vi "LEBITplc.ParseMin&MaxArray.vi"(2 "Min&MaxArray":string[][](array[string])) -> (15 "MinSetValue":dbl[](array[numeric]), 16 "MaxSetValue":dbl[](array[numeric]), 17 "SetValueInfoServiceId":i32[](array[numeric]))   [LabVIEW 2014, in "LEBITplc.lvlib"]
uses:
  LEBITplc.lvlib
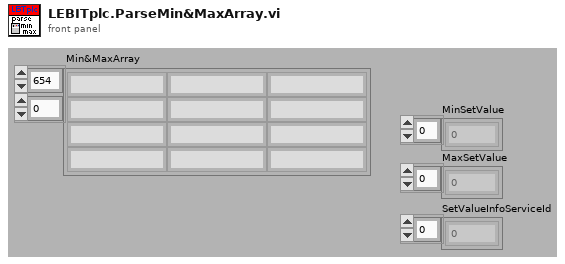
[diagram p1: front panel]
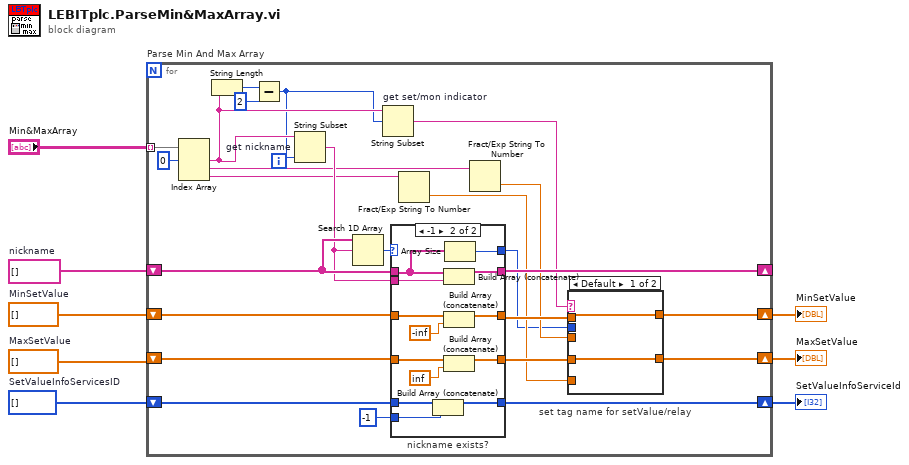
[diagram p0: block diagram]
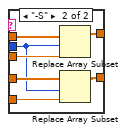
[diagram p3: hidden frame]
diagram:
  w4 = i32[] []  # SetValueInfoServicesID
  w5 = dbl[] []  # MaxSetValue
  w6 = dbl[] []  # MinSetValue
  w8 = string[] []  # nickname
  n1 = for "Parse Min And Max Array" {
    tunnel: "Min&MaxArray" -> [w33] mode=indexing
    shift-right: [w22] -> _
    shift-left: w8 -> [w26]
    shift-right: [w21] -> w2
    shift-left: w5 -> [w13]
    shift-right: [w10] -> w1
    shift-left: w4 -> [w20]
    shift-right: [w12] -> w3
    shift-left: w6 -> [w18]
    n2 = Index Array(array=w33, index #1=0 ("index")) -> (element #1=w29:string, element #2=w17:string, element #3=w16:string)  [unwired: 2 in]
    n3 = String Length(string=w29) -> (length=w31:i32)
    n4 = Subtract(x=w31, y=2) -> (x-y=w28:i32)
    n5 = String Subset "get nickname"(string=w29, length (rest)=w28) -> (substring=w25:string)  [unwired: 1 in]
    n6 = Search 1D Array(1D array=w26, element=w25) -> (index of element=w27:i32)  [unwired: 1 in]
    n7 = String Subset "get set/mon indicator"(string=w29, offset (0)=w28) -> (substring=w19:string)  [unwired: 1 in]
    n8 = case "nickname exists?" shown="-1" w27 {
      selector: w27 -> [w35 _]
      tunnel: w26 -> [w38 w44]
      tunnel: w25 -> [_ w51]
      tunnel: [w38 w50] -> w22
      tunnel: w13 -> [w37 w49]
      tunnel: w20 -> [w36 w48]
      tunnel: [w34 w47] -> w24
      tunnel: [w37 w46] -> w23
      tunnel: [w36 w45] -> w10
      tunnel: [w35 w43] -> w9
      tunnel: w18 -> [w34 w42]
      tunnel: -1 -> [_ w39]
      frame 0, Default {
      }
      frame -1 {
        n9 = Build Array (concatenate)(w48, w39) -> (w45:i32[])
        n10 = Build Array (concatenate)(w44, w51) -> (w50:string[])
        n11 = Build Array (concatenate)(w42, -inf) -> (w47:dbl[])
        n12 = Build Array (concatenate)(w49, inf) -> (w46:dbl[])
        n13 = Array Size(array=w44) -> (size(s)=w43:i32)
      }
    }
    n14 = Fract/Exp String To Number(string=w16) -> (number=w14:dbl)  [unwired: 3 in, 1 out]
    n15 = Fract/Exp String To Number(string=w17) -> (number=w15:dbl)  [unwired: 3 in, 1 out]
    n16 = case "set tag name for setValue/relay" shown="Default" w19 {
      tunnel: w24 -> [w53 w60]
      tunnel: w9 -> [_ w54]
      tunnel: w15 -> [_ w59]
      tunnel: w23 -> [w52 w56]
      tunnel: w14 -> [_ w55]
      tunnel: [w53 w58] -> w12
      tunnel: [w52 w57] -> w21
      frame Default {
      }
      frame "-S" {
        n17 = Replace Array Subset(array=w60, new element=w59, index=w54) -> (w58:dbl[])
        n18 = Replace Array Subset(array=w56, new element=w55, index=w54) -> (w57:dbl[])
      }
    }
  }
  "MinSetValue" <- w3
  "MaxSetValue" <- w2
  "SetValueInfoServiceId" <- w1
